vi "PP.Create.File.By.ByteArray.vi"(7 "u8 Data[]":u8[](array[numeric]) format="%.0x", 8 "error in":errorcluster, 11 "file path (use dialog)":path) -> (0 "error out":errorcluster, 3 "file path out":path)   [LabVIEW 2020, in "PixPack.lvlib"]
uses:
  PixPack.lvlib
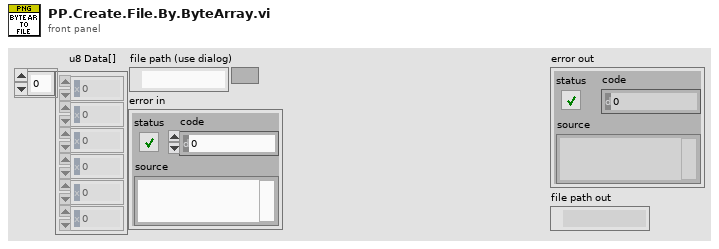
[diagram p1: front panel]
types:
  T1 = enum16{"big-endian, network order", "native, host order", "little-endian"}
  T2 = enum16{"open", "replace", "create", "open or create", "replace or create", "replace or create with confirmation"}
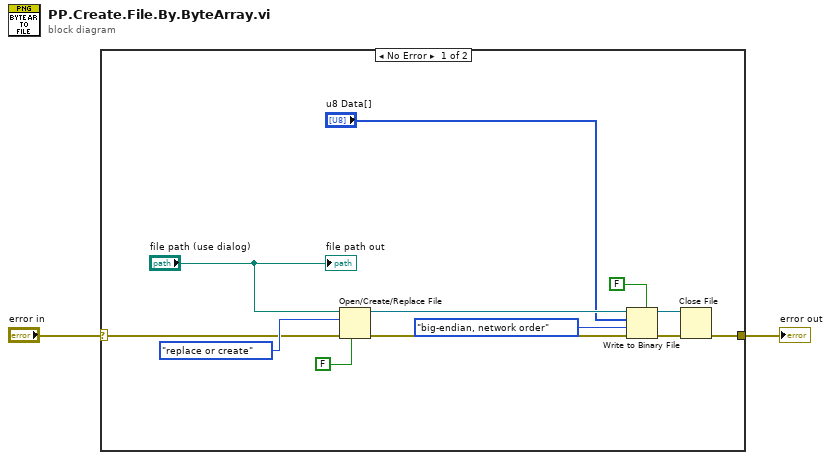
[diagram p0: block diagram]
diagram:
  n1 = case shown="No Error" "error in" {
    selector: "error in" -> [w4 w15]
    tunnel: [w3 w15] -> w1
    frame No Error {
      n2 = Open/Create/Replace File(file path (use dialog)="file path (use dialog)", error in=w4, operation (0:open)=T2."replace or create", disable buffering (F)=FALSE) -> (refnum out=w7:refnum<file>, error out=w9:errorcluster)  [unwired: 2 in, 1 out]
      n3 = Write to Binary File(file (use dialog)=w7, data="u8 Data[]", error in=w9, 5:FALSE ("prepend array or string size? (T)"), 9:T1."big-endian, network order" ("byte order (0:big-endian, network order)")) -> (refnum out=w12:refnum<file>, error out=w11:errorcluster)  [unwired: 1 in, 1 out]
      n4 = Close File(refnum=w12, error in=w11) -> (error out=w3:errorcluster)  [unwired: 1 out]
      "file path out" <- "file path (use dialog)"
    }
    frame Error {
    }
  }
  "error out" <- w1
